vi "HFRR ADV v026 new software.vi"() -> ()   [LabVIEW 2025] (continued)
                n1899 = local read "string1"() -> (w2377:string)
              }
              frame True {
                n1900 = local read "String Indicator 4"() -> (w2378:string)
              }
            }
            n1901 = local read "string1 3"() -> (w2275:string)
            n1902 = String To Path(string=w2231) -> (path=w2362:path)
            n1903 = String To Path(string=w2275) -> (path=w2373:path)
            n1904 = local read "Numeric 12"() -> (w2359:i32)
            n1905 = local read "Numeric 8"() -> (w2361:i32)
            n1906 = local read "string1 2"() -> (w2276:string)
            n1907 = local read "string1 4"() -> (w2274:string)
            n1908 = Open/Create/Replace File "Open File"(file path (use dialog)=w2362) -> (refnum out=w2376:refnum<file>, error out=w2375:errorcluster)  [unwired: 5 in, 1 out]
            n1909 = Open/Create/Replace File "Open File"(file path (use dialog)=w2373) -> (refnum out=w2369:refnum<file>, error out=w2370:errorcluster)  [unwired: 5 in, 1 out]
            n1910 = for {
              N: w2361 -> [_]
              tunnel: w2376 -> [w2524]
              tunnel: w2375 -> [w2523]
              tunnel: [w2513] -> w2288 mode=indexing
              tunnel: [w2511] -> w2345 mode=indexing
              tunnel: [w2512] -> w2340 mode=indexing
              tunnel: w2357 -> [_]
              tunnel: [w2505] -> w2342 mode=indexing
              tunnel: [w2501] -> w2311 mode=indexing
              tunnel: [w2497] -> w2286 mode=indexing
              tunnel: [w2493] -> w2267 mode=indexing
              tunnel: [w2488] -> w2227 mode=indexing
              (unwired) TRUE ("line mode (F)")
              # "freq"
              # "Stroke"
              # "Time"
              # "CoF"
              # "Humidity"
              # "Temp"
              # "Air Temp"
              # "ECR"
              n1911 = Read from Text File "Read File"(file (use dialog)=w2524, error in=w2523) -> (text=w2489:string)  [unwired: 2 in, 3 out]
              n1912 = local write "String 6"(w2489) -> ()
              n1913 = String Subset(string=w2489, offset (0)=0, length (rest)=14 ("length (rest)")) -> (substring=w2517:string)
              n1914 = String Subset(string=w2489, offset (0)=35, length (rest)=9 ("length (rest)")) -> (substring=w2514:string)
              n1915 = String Subset(string=w2489, offset (0)=15, length (rest)=9 ("length (rest)")) -> (substring=w2520:string)
              n1916 = Fract/Exp String To Number(string=w2517) -> (number=w2513:dbl)  [unwired: 3 in, 1 out]
              n1917 = Fract/Exp String To Number(string=w2514) -> (number=w2512:dbl)  [unwired: 3 in, 1 out]
              n1918 = Fract/Exp String To Number(string=w2520) -> (number=w2511:dbl)  [unwired: 3 in, 1 out]
              n1919 = String Subset(string=w2489, offset (0)=85, length (rest)=9 ("length (rest)")) -> (substring=w2490:string)
              n1920 = String Subset(string=w2489, offset (0)=25, length (rest)=9 ("length (rest)")) -> (substring=w2496:string)
              n1921 = String Subset(string=w2489, offset (0)=55, length (rest)=9 ("length (rest)")) -> (substring=w2498:string)
              n1922 = String Subset(string=w2489, offset (0)=45, length (rest)=9 ("length (rest)")) -> (substring=w2504:string)
              n1923 = String Subset(string=w2489, offset (0)=65, length (rest)=9 ("length (rest)")) -> (substring=w2510:string)
              n1924 = Fract/Exp String To Number(string=w2496) -> (number=w2493:dbl)  [unwired: 3 in, 1 out]
              n1925 = Fract/Exp String To Number(string=w2490) -> (number=w2488:dbl)  [unwired: 3 in, 1 out]
              n1926 = Fract/Exp String To Number(string=w2498) -> (number=w2497:dbl)  [unwired: 3 in, 1 out]
              n1927 = Fract/Exp String To Number(string=w2504) -> (number=w2501:dbl)  [unwired: 3 in, 1 out]
              n1928 = Fract/Exp String To Number(string=w2510) -> (number=w2507:dbl)  [unwired: 3 in, 1 out]
              n1929 = Add(x=w2507, y=0.0) -> (x+y=w2505:dbl)
            }
            n1930 = for {
              N: w2359 -> [_]
              tunnel: w2370 -> [w2450]
              tunnel: w2369 -> [w2449]
              tunnel: [w2439] -> w2328 mode=indexing
              tunnel: [w2437] -> w2326 mode=indexing
              tunnel: [w2438] -> w2322 mode=indexing
              tunnel: w2357 -> [_]
              tunnel: [w2431] -> w2324 mode=indexing
              tunnel: [w2427] -> w2306 mode=indexing
              tunnel: [w2423] -> w2282 mode=indexing
              tunnel: [w2420] -> w2263 mode=indexing
              tunnel: [w2416] -> w2222 mode=indexing
              (unwired) 9 ("length (rest)")
              (unwired) 9 ("length (rest)")
              (unwired) TRUE ("line mode (F)")
              n1931 = Read from Text File "Read File"(file (use dialog)=w2449, error in=w2450) -> (text=w2417:string)  [unwired: 2 in, 3 out]
              n1932 = local write "String 8"(w2417) -> ()
              n1933 = String Subset(string=w2417, offset (0)=85) -> (substring=w2419:string)  [unwired: 1 in]
              n1934 = String Subset(string=w2417, offset (0)=35, length (rest)=9 ("length (rest)")) -> (substring=w2440:string)
              n1935 = String Subset(string=w2417, offset (0)=55, length (rest)=9 ("length (rest)")) -> (substring=w2425:string)
              n1936 = String Subset(string=w2417, offset (0)=25) -> (substring=w2421:string)  [unwired: 1 in]
              n1937 = String Subset(string=w2417, offset (0)=15, length (rest)=9 ("length (rest)")) -> (substring=w2446:string)
              n1938 = String Subset(string=w2417, offset (0)=0, length (rest)=14 ("length (rest)")) -> (substring=w2443:string)
              n1939 = String Subset(string=w2417, offset (0)=45, length (rest)=9 ("length (rest)")) -> (substring=w2430:string)
              n1940 = String Subset(string=w2417, offset (0)=65, length (rest)=9 ("length (rest)")) -> (substring=w2436:string)
              n1941 = Fract/Exp String To Number(string=w2419) -> (number=w2416:dbl)  [unwired: 3 in, 1 out]
              n1942 = Fract/Exp String To Number(string=w2440) -> (number=w2438:dbl)  [unwired: 3 in, 1 out]
              n1943 = Fract/Exp String To Number(string=w2425) -> (number=w2423:dbl)  [unwired: 3 in, 1 out]
              n1944 = Fract/Exp String To Number(string=w2421) -> (number=w2420:dbl)  [unwired: 3 in, 1 out]
              n1945 = Fract/Exp String To Number(string=w2446) -> (number=w2437:dbl)  [unwired: 3 in, 1 out]
              n1946 = Fract/Exp String To Number(string=w2443) -> (number=w2439:dbl)  [unwired: 3 in, 1 out]
              n1947 = Fract/Exp String To Number(string=w2430) -> (number=w2427:dbl)  [unwired: 3 in, 1 out]
              n1948 = Fract/Exp String To Number(string=w2436) -> (number=w2433:dbl)  [unwired: 3 in, 1 out]
              n1949 = Add(x=w2433, y=0.0) -> (x+y=w2431:dbl)
            }
            n1950 = String To Path(string=w2276) -> (path=w2374:path)
            n1951 = String To Path(string=w2274) -> (path=w2368:path)
            n1952 = local read "Numeric 11"() -> (w2358:i32)
            n1953 = local read "Numeric 13"() -> (w2360:i32)
            n1954 = Open/Create/Replace File "Open File"(file path (use dialog)=w2374) -> (refnum out=w2372:refnum<file>, error out=w2371:errorcluster)  [unwired: 5 in, 1 out]
            n1955 = Open/Create/Replace File "Open File"(file path (use dialog)=w2368) -> (refnum out=w2367:refnum<file>, error out=w2366:errorcluster)  [unwired: 5 in, 1 out]
            n1956 = for {
              N: w2358 -> [_]
              tunnel: w2372 -> [w2487]
              tunnel: w2371 -> [w2486]
              tunnel: [w2476] -> w2338 mode=indexing
              tunnel: [w2474] -> w2336 mode=indexing
              tunnel: [w2475] -> w2331 mode=indexing
              tunnel: w2357 -> [_]
              tunnel: [w2468] -> w2333 mode=indexing
              tunnel: [w2464] -> w2309 mode=indexing
              tunnel: [w2460] -> w2284 mode=indexing
              tunnel: [w2456] -> w2265 mode=indexing
              tunnel: [w2451] -> w2223 mode=indexing
              (unwired) TRUE ("line mode (F)")
              n1957 = Read from Text File "Read File"(file (use dialog)=w2487, error in=w2486) -> (text=w2452:string)  [unwired: 2 in, 3 out]
              n1958 = local write "String 7"(w2452) -> ()
              n1959 = String Subset(string=w2452, offset (0)=85, length (rest)=9 ("length (rest)")) -> (substring=w2455:string)
              n1960 = String Subset(string=w2452, offset (0)=35, length (rest)=9 ("length (rest)")) -> (substring=w2477:string)
              n1961 = String Subset(string=w2452, offset (0)=55, length (rest)=9 ("length (rest)")) -> (substring=w2463:string)
              n1962 = String Subset(string=w2452, offset (0)=25, length (rest)=9 ("length (rest)")) -> (substring=w2457:string)
              n1963 = String Subset(string=w2452, offset (0)=45, length (rest)=9 ("length (rest)")) -> (substring=w2465:string)
              n1964 = String Subset(string=w2452, offset (0)=0, length (rest)=14 ("length (rest)")) -> (substring=w2480:string)
              n1965 = String Subset(string=w2452, offset (0)=15, length (rest)=9 ("length (rest)")) -> (substring=w2483:string)
              n1966 = String Subset(string=w2452, offset (0)=65, length (rest)=9 ("length (rest)")) -> (substring=w2469:string)
              n1967 = Fract/Exp String To Number(string=w2455) -> (number=w2451:dbl)  [unwired: 3 in, 1 out]
              n1968 = Fract/Exp String To Number(string=w2477) -> (number=w2475:dbl)  [unwired: 3 in, 1 out]
              n1969 = Fract/Exp String To Number(string=w2463) -> (number=w2460:dbl)  [unwired: 3 in, 1 out]
              n1970 = Fract/Exp String To Number(string=w2457) -> (number=w2456:dbl)  [unwired: 3 in, 1 out]
              n1971 = Fract/Exp String To Number(string=w2465) -> (number=w2464:dbl)  [unwired: 3 in, 1 out]
              n1972 = Fract/Exp String To Number(string=w2480) -> (number=w2476:dbl)  [unwired: 3 in, 1 out]
              n1973 = Fract/Exp String To Number(string=w2483) -> (number=w2474:dbl)  [unwired: 3 in, 1 out]
              n1974 = Fract/Exp String To Number(string=w2469) -> (number=w2472:dbl)  [unwired: 3 in, 1 out]
              n1975 = Add(x=w2472, y=0.0) -> (x+y=w2468:dbl)
            }
            n1976 = for {
              N: w2360 -> [_]
              tunnel: w2367 -> [w2415]
              tunnel: w2366 -> [w2414]
              tunnel: [w2404] -> w2320 mode=indexing
              tunnel: [w2403] -> w2313 mode=indexing
              tunnel: w2357 -> [_]
              tunnel: [w2392] -> w2318 mode=indexing
              tunnel: [w2397] -> w2315 mode=indexing
              tunnel: [w2393] -> w2305 mode=indexing
              tunnel: [w2388] -> w2280 mode=indexing
              tunnel: [w2384] -> w2261 mode=indexing
              tunnel: [w2379] -> w2221 mode=indexing
              (unwired) 1.0 ("x")
              (unwired) TRUE ("line mode (F)")
              n1977 = Read from Text File "Read File"(file (use dialog)=w2415, error in=w2414) -> (text=w2380:string)  [unwired: 2 in, 3 out]
              n1978 = local write "String 12"(w2380) -> ()
              n1979 = String Subset(string=w2380, offset (0)=85, length (rest)=9 ("length (rest)")) -> (substring=w2382:string)
              n1980 = String Subset(string=w2380, offset (0)=35, length (rest)=9 ("length (rest)")) -> (substring=w2405:string)
              n1981 = String Subset(string=w2380, offset (0)=55, length (rest)=9 ("length (rest)")) -> (substring=w2390:string)
              n1982 = String Subset(string=w2380, offset (0)=25, length (rest)=9 ("length (rest)")) -> (substring=w2386:string)
              n1983 = String Subset(string=w2380, offset (0)=45, length (rest)=9 ("length (rest)")) -> (substring=w2395:string)
              n1984 = String Subset(string=w2380, offset (0)=15, length (rest)=9 ("length (rest)")) -> (substring=w2411:string)
              n1985 = String Subset(string=w2380, offset (0)=0, length (rest)=14 ("length (rest)")) -> (substring=w2408:string)
              n1986 = String Subset(string=w2380, offset (0)=65, length (rest)=9 ("length (rest)")) -> (substring=w2398:string)
              n1987 = Fract/Exp String To Number(string=w2382) -> (number=w2379:dbl)  [unwired: 3 in, 1 out]
              n1988 = Fract/Exp String To Number(string=w2405) -> (number=w2403:dbl)  [unwired: 3 in, 1 out]
              n1989 = Fract/Exp String To Number(string=w2390) -> (number=w2388:dbl)  [unwired: 3 in, 1 out]
              n1990 = Fract/Exp String To Number(string=w2386) -> (number=w2384:dbl)  [unwired: 3 in, 1 out]
              n1991 = Fract/Exp String To Number(string=w2395) -> (number=w2393:dbl)  [unwired: 3 in, 1 out]
              n1992 = Fract/Exp String To Number(string=w2411) -> (number=w2392:dbl)  [unwired: 3 in, 1 out]
              n1993 = Fract/Exp String To Number(string=w2408) -> (number=w2404:dbl)  [unwired: 3 in, 1 out]
              n1994 = Fract/Exp String To Number(string=w2398) -> (number=w2401:dbl)  [unwired: 3 in, 1 out]
              n1995 = Add(x=w2401, y=0.0) -> (x+y=w2397:dbl)
            }
            n1996 = Delete From Array(array=w2263, index=0) -> (array with subset deleted=w2236:dbl[])  [unwired: 1 in, 1 out]
            n1997 = Delete From Array(array=w2326, index=0) -> (array with subset deleted=w2299:dbl[])  [unwired: 1 in, 1 out]
            n1998 = Delete From Array(array=w2306, index=0) -> (array with subset deleted=w2294:dbl[])  [unwired: 1 in, 1 out]
            n1999 = Delete From Array(array=w2324, index=0) -> (array with subset deleted=w2325:dbl[])  [unwired: 1 in, 1 out]
            n2000 = call-poly <vilib>:"Mean.vi"("X"=w2236) -> ("mean"=→"КОФ2 4":dbl)  [unwired: 1 out]
            n2001 = call-poly <vilib>:"Mean.vi"("X"=w2299) -> ("mean"=→"КОФ3":dbl)  [unwired: 1 out]
            n2002 = call-poly <vilib>:"Mean.vi"("X"=w2294) -> ("mean"=→"CP3":dbl)  [unwired: 1 out]
            n2003 = Delete From Array(array=w2288, index=0) -> (array with subset deleted=w2215:dbl[])  [unwired: 1 in, 1 out]
            n2004 = Delete From Array(array=w2227, index=0) -> (array with subset deleted=w2214:dbl[])  [unwired: 1 in, 1 out]
            n2005 = Delete From Array(array=w2267, index=0) -> (array with subset deleted=w2238:dbl[])  [unwired: 1 in, 1 out]
            n2006 = Delete From Array(array=w2345, index=0) -> (array with subset deleted=w2300:dbl[])  [unwired: 1 in, 1 out]
            n2007 = Delete From Array(array=w2311, index=0) -> (array with subset deleted=w2296:dbl[])  [unwired: 1 in, 1 out]
            "array w/ subset deleted" <- w2296
            n2008 = Delete From Array(array=w2342, index=0) -> (array with subset deleted=w2343:dbl[])  [unwired: 1 in, 1 out]
            n2009 = call-poly <vilib>:"Mean.vi"("X"=w2238) -> ("mean"=→"КОФ2 2":dbl)  [unwired: 1 out]
            n2010 = call-poly <vilib>:"Mean.vi"("X"=w2300) -> ("mean"=→"КОФ1":dbl)  [unwired: 1 out]
            n2011 = Bundle "Bundle"(w2215, w2214) -> (w2220:cluster{dbl[], dbl[]})  [unwired: 1 in]
            n2012 = Bundle "Bundle"(w2215, w2343) -> (w2207:cluster{dbl[], dbl[]})  [unwired: 1 in]
            n2013 = Delete From Array(array=w2222, index=0) -> (array with subset deleted=w2210:dbl[])  [unwired: 1 in, 1 out]
            n2014 = Delete From Array(array=w2223, index=0) -> (array with subset deleted=w2212:dbl[])  [unwired: 1 in, 1 out]
            n2015 = Delete From Array(array=w2333, index=0) -> (array with subset deleted=w2334:dbl[])  [unwired: 1 in, 1 out]
            n2016 = Delete From Array(array=w2221, index=0) -> (array with subset deleted=w2208:dbl[])  [unwired: 1 in, 1 out]
            n2017 = Delete From Array(array=w2315, index=0) -> (array with subset deleted=w2316:dbl[])  [unwired: 1 in, 1 out]
            n2018 = Delete From Array(array=w2340, index=0) -> (array with subset deleted=w2246:dbl[])  [unwired: 1 in, 1 out]
            n2019 = Delete From Array(array=w2286, index=0) -> (array with subset deleted=w2242:dbl[])  [unwired: 1 in, 1 out]
            n2020 = Delete From Array(array=w2322, index=0) -> (array with subset deleted=w2244:dbl[])  [unwired: 1 in, 1 out]
            n2021 = Delete From Array(array=w2282, index=0) -> (array with subset deleted=w2240:dbl[])  [unwired: 1 in, 1 out]
            n2022 = Delete From Array(array=w2331, index=0) -> (array with subset deleted=w2245:dbl[])  [unwired: 1 in, 1 out]
            n2023 = Delete From Array(array=w2284, index=0) -> (array with subset deleted=w2241:dbl[])  [unwired: 1 in, 1 out]
            n2024 = Delete From Array(array=w2265, index=0) -> (array with subset deleted=w2237:dbl[])  [unwired: 1 in, 1 out]
            n2025 = Delete From Array(array=w2309, index=0) -> (array with subset deleted=w2295:dbl[])  [unwired: 1 in, 1 out]
            n2026 = Delete From Array(array=w2336, index=0) -> (array with subset deleted=w2297:dbl[])  [unwired: 1 in, 1 out]
            n2027 = Delete From Array(array=w2313, index=0) -> (array with subset deleted=w2243:dbl[])  [unwired: 1 in, 1 out]
            n2028 = Delete From Array(array=w2280, index=0) -> (array with subset deleted=w2239:dbl[])  [unwired: 1 in, 1 out]
            n2029 = Delete From Array(array=w2261, index=0) -> (array with subset deleted=w2235:dbl[])  [unwired: 1 in, 1 out]
            n2030 = Delete From Array(array=w2305, index=0) -> (array with subset deleted=w2293:dbl[])  [unwired: 1 in, 1 out]
            n2031 = Delete From Array(array=w2318, index=0) -> (array with subset deleted=w2298:dbl[])  [unwired: 1 in, 1 out]
            n2032 = Delete From Array(array=w2328, index=0) -> (array with subset deleted=w2211:dbl[])  [unwired: 1 in, 1 out]
            n2033 = Delete From Array(array=w2338, index=0) -> (array with subset deleted=w2213:dbl[])  [unwired: 1 in, 1 out]
            n2034 = Delete From Array(array=w2320, index=0) -> (array with subset deleted=w2209:dbl[])  [unwired: 1 in, 1 out]
            n2035 = Bundle "Bundle"(w2215, w2246) -> (w2233:cluster{dbl[], dbl[]})  [unwired: 1 in]
            n2036 = Bundle "Bundle"(w2215, w2300) -> (w2234:cluster{dbl[], dbl[]})  [unwired: 1 in]
            n2037 = Bundle "Bundle"(w2246, w2242) -> (w2248:cluster{dbl[], dbl[]})  [unwired: 1 in]
            n2038 = Bundle "Bundle"(w2211, w2210) -> (w2218:cluster{dbl[], dbl[]})  [unwired: 1 in]
            n2039 = Bundle "Bundle"(w2244, w2240) -> (w2250:cluster{dbl[], dbl[]})  [unwired: 1 in]
            n2040 = Bundle "Bundle"(w2211, w2244) -> (w2354:cluster{dbl[], dbl[]})  [unwired: 1 in]
            n2041 = Bundle "Bundle"(w2211, w2240) -> (w2278:cluster{dbl[], dbl[]})  [unwired: 1 in]
            n2042 = Bundle "Bundle"(w2211, w2299) -> (w2364:cluster{dbl[], dbl[]})  [unwired: 1 in]
            n2043 = Bundle "Bundle"(w2211, w2294) -> (w2302:cluster{dbl[], dbl[]})  [unwired: 1 in]
            n2044 = Bundle "Bundle"(w2211, w2325) -> (w2349:cluster{dbl[], dbl[]})  [unwired: 1 in]
            n2045 = Bundle "Bundle"(w2245, w2241) -> (w2249:cluster{dbl[], dbl[]})  [unwired: 1 in]
            n2046 = Bundle "Bundle"(w2213, w2212) -> (w2219:cluster{dbl[], dbl[]})  [unwired: 1 in]
            n2047 = Bundle "Bundle"(w2213, w2245) -> (w2356:cluster{dbl[], dbl[]})  [unwired: 1 in]
            n2048 = Bundle "Bundle"(w2213, w2241) -> (w2279:cluster{dbl[], dbl[]})  [unwired: 1 in]
            n2049 = Bundle "Bundle"(w2213, w2295) -> (w2303:cluster{dbl[], dbl[]})  [unwired: 1 in]
            n2050 = Bundle "Bundle"(w2213, w2297) -> (w2365:cluster{dbl[], dbl[]})  [unwired: 1 in]
            n2051 = Bundle "Bundle"(w2213, w2334) -> (w2347:cluster{dbl[], dbl[]})  [unwired: 1 in]
            n2052 = Bundle "Bundle"(w2243, w2239) -> (w2251:cluster{dbl[], dbl[]})  [unwired: 1 in]
            n2053 = Bundle "Bundle"(w2209, w2208) -> (w2217:cluster{dbl[], dbl[]})  [unwired: 1 in]
            n2054 = Bundle "Bundle"(w2209, w2243) -> (w2355:cluster{dbl[], dbl[]})  [unwired: 1 in]
            n2055 = Bundle "Bundle"(w2209, w2239) -> (w2277:cluster{dbl[], dbl[]})  [unwired: 1 in]
            n2056 = Bundle "Bundle"(w2209, w2293) -> (w2301:cluster{dbl[], dbl[]})  [unwired: 1 in]
            n2057 = Bundle "Bundle"(w2209, w2298) -> (w2363:cluster{dbl[], dbl[]})  [unwired: 1 in]
            n2058 = Bundle "Bundle"(w2209, w2316) -> (w2348:cluster{dbl[], dbl[]})  [unwired: 1 in]
            n2059 = call-poly <vilib>:"Mean.vi"("X"=w2296) -> ("mean"=→"CP1":dbl)  [unwired: 1 out]
            n2060 = call-poly <vilib>:"Mean.vi"("X"=w2237) -> ("mean"=→"КОФ2 3":dbl)  [unwired: 1 out]
            n2061 = call-poly <vilib>:"Mean.vi"("X"=w2295) -> ("mean"=→"CP2":dbl)  [unwired: 1 out]
            n2062 = call-poly <vilib>:"Mean.vi"("X"=w2297) -> ("mean"=→"КОФ2":dbl)  [unwired: 1 out]
            n2063 = call-poly <vilib>:"Mean.vi"("X"=w2235) -> ("mean"=→"КОФ2 5":dbl)  [unwired: 1 out]
            n2064 = call-poly <vilib>:"Mean.vi"("X"=w2293) -> ("mean"=→"CP4":dbl)  [unwired: 1 out]
            n2065 = call-poly <vilib>:"Mean.vi"("X"=w2298) -> ("mean"=→"КОФ4":dbl)  [unwired: 1 out]
            n2066 = Bundle "Bundle"(w2215, w2242) -> (w2206:cluster{dbl[], dbl[]})  [unwired: 1 in]
            n2067 = Bundle "Bundle"(w2215, w2296) -> (w2229:cluster{dbl[], dbl[]})  [unwired: 1 in]
            n2068 = Build Array "Build Array"(w2206, w2229) -> (w2232:cluster{dbl[], dbl[]}[])
            "XY Graph 17" <- w2232
            n2069 = Build Array "Build Array"(w2220, w2219, w2218, w2217) -> (→"Frequency ( Hz )":cluster{dbl[], dbl[]}[])
            n2070 = Build Array "Build Array"(w2248, w2249, w2250, w2251) -> (→"Air Temp ( °C ) vs Humidity ( % RH )":cluster{dbl[], dbl[]}[])
            n2071 = Build Array "Build Array"(w2233, w2356, w2354, w2355) -> (→"Air Temperature  ( °C )":cluster{dbl[], dbl[]}[])
            n2072 = Build Array "Build Array"(w2206, w2279, w2278, w2277) -> (→"Humidity ( %RH )":cluster{dbl[], dbl[]}[])
            n2073 = Build Array "Build Array"(w2234, w2365, w2364, w2363) -> (→"Coefficient Of Friction":cluster{dbl[], dbl[]}[])
            n2074 = Build Array "Build Array"(w2229, w2303, w2302, w2301) -> (→"Sample Temperature ( °C )":cluster{dbl[], dbl[]}[])
            n2075 = Build Array "Build Array"(w2207, w2347, w2349, w2348) -> (→"XY Graph 13":cluster{dbl[], dbl[]}[])
            n2076 = Bundle "Bundle"(w2215, w2238) -> (w2260:cluster{dbl[], dbl[]})  [unwired: 1 in]
            n2077 = Bundle "Bundle"(w2211, w2236) -> (w2258:cluster{dbl[], dbl[]})  [unwired: 1 in]
            n2078 = Bundle "Bundle"(w2213, w2237) -> (w2259:cluster{dbl[], dbl[]})  [unwired: 1 in]
            n2079 = Bundle "Bundle"(w2209, w2235) -> (w2257:cluster{dbl[], dbl[]})  [unwired: 1 in]
            n2080 = Build Array "Build Array"(w2260, w2259, w2258, w2257) -> (→"Stroke ( mm )":cluster{dbl[], dbl[]}[])
            n2081 = local write "XY Graph 16"(w2232) -> ()
          }
          frame #2 {
          }
          frame #3 {
            n2082 = local write "Numeric 8"(0 ("Numeric 8")) -> ()
            n2083 = local write "Numeric 11"(0 ("Numeric 11")) -> ()
            n2084 = local write "Numeric 12"(0 ("Numeric 12")) -> ()
            n2085 = local write "Numeric 13"(0 ("Numeric 13")) -> ()
            n2086 = property on="OPEN" class="Bool (strict)"("Visible"=TRUE) -> ()  [unwired: 2 in, 2 out]
            n2087 = local read "String Control 2"() -> (w2532:string)
            n2088 = local read "String Control 4"() -> (w2531:string)
            n2089 = local read "String Control 6"() -> (w2530:string)
            n2090 = local read "String Control 8"() -> (w2529:string)
            n2091 = Match Pattern(string=w2532, regular expression="Samples / cycle :- ") -> (after substring=w2546:string)  [unwired: 1 in, 3 out]
            n2092 = Match Pattern(string=w2532, regular expression="Frequency :- ") -> (after substring=w2565:string)  [unwired: 1 in, 3 out]
            n2093 = Match Pattern(string=w2531, regular expression="Samples / cycle :- ") -> (after substring=w2542:string)  [unwired: 1 in, 3 out]
            n2094 = Match Pattern(string=w2531, regular expression="Frequency :- ") -> (after substring=w2560:string)  [unwired: 1 in, 3 out]
            n2095 = Match Pattern(string=w2530, regular expression="Samples / cycle :- ") -> (after substring=w2538:string)  [unwired: 1 in, 3 out]
            n2096 = Match Pattern(string=w2530, regular expression="Frequency :- ") -> (after substring=w2555:string)  [unwired: 1 in, 3 out]
            n2097 = Match Pattern(string=w2529, regular expression="Samples / cycle :- ") -> (after substring=w2534:string)  [unwired: 1 in, 3 out]
            n2098 = Match Pattern(string=w2529, regular expression="Frequency :- ") -> (after substring=w2550:string)  [unwired: 1 in, 3 out]
            n2099 = String Subset(string=w2546, length (rest)=6 ("length (rest)")) -> (substring=w2548:string)  [unwired: 1 in]
            n2100 = String Subset(string=w2565, length (rest)=9 ("length (rest)")) -> (substring=w2567:string)  [unwired: 1 in]
            n2101 = String Subset(string=w2542, length (rest)=6 ("length (rest)")) -> (substring=w2544:string)  [unwired: 1 in]
            n2102 = String Subset(string=w2560, length (rest)=9 ("length (rest)")) -> (substring=w2562:string)  [unwired: 1 in]
            n2103 = String Subset(string=w2538, length (rest)=6 ("length (rest)")) -> (substring=w2540:string)  [unwired: 1 in]
            n2104 = String Subset(string=w2555, length (rest)=9 ("length (rest)")) -> (substring=w2557:string)  [unwired: 1 in]
            n2105 = String Subset(string=w2534, length (rest)=6 ("length (rest)")) -> (substring=w2536:string)  [unwired: 1 in]
            n2106 = String Subset(string=w2550, length (rest)=9 ("length (rest)")) -> (substring=w2552:string)  [unwired: 1 in]
            n2107 = Fract/Exp String To Number(string=w2548) -> (number=w2528:dbl)  [unwired: 3 in, 1 out]
            n2108 = Fract/Exp String To Number(string=w2567) -> (number=w2568:dbl)  [unwired: 3 in, 1 out]
            n2109 = Fract/Exp String To Number(string=w2544) -> (number=w2527:dbl)  [unwired: 3 in, 1 out]
            n2110 = Fract/Exp String To Number(string=w2562) -> (number=w2563:dbl)  [unwired: 3 in, 1 out]
            n2111 = Fract/Exp String To Number(string=w2540) -> (number=w2526:dbl)  [unwired: 3 in, 1 out]
            n2112 = Fract/Exp String To Number(string=w2557) -> (number=w2558:dbl)  [unwired: 3 in, 1 out]
            n2113 = Fract/Exp String To Number(string=w2536) -> (number=w2525:dbl)  [unwired: 3 in, 1 out]
            n2114 = Fract/Exp String To Number(string=w2552) -> (number=w2553:dbl)  [unwired: 3 in, 1 out]
            n2115 = local write "sample1"(w2528) -> ()
            n2116 = local write "freq1"(w2568) -> ()
            n2117 = local write "sample2"(w2527) -> ()
            n2118 = local write "freq2"(w2563) -> ()
            n2119 = local write "sample3"(w2526) -> ()
            n2120 = local write "freq3"(w2558) -> ()
            n2121 = local write "sample4"(w2525) -> ()
            n2122 = local write "freq 4"(w2553) -> ()
          }
        }
      }
    }
    n2123 = case shown="True" w2126 {
      selector: w2126 -> [_ w2145]
      frame False {
      }
      frame True {
        n2124 = Not(x=w2145) -> (.not. x?=w2141:bool)
        n2125 = local write "service 3"(w2141) -> ()
        n2126 = local write "OPEN 6"(w2141) -> ()
        n2127 = call <vilib>:"System Exec.vi"("wait until completion? (T)"=TRUE, "command line"="C:\\LAB-IQ\\Scar View.exe") -> ("error out"=→"error out 5":errorcluster)  [unwired: 6 in, 3 out]
      }
    }
    n2128 = case shown="\"Acquire\", Default" w2135 {
      frame "Acquire", Default {
        # "Elapsed time\ncof\nstroke\nAir temp\nTemp\nHumidity"
        n2129 = disable-structure shown="Disabled" {
          frame Disabled {
            n2130 = local read "Flag"() -> (w2844:dbl)
            n2131 = local read "RUN"() -> (w2841:bool)
            n2132 = Not(x=w2841) -> (.not. x?=w2840:bool)
            n2133 = Equal?(x=w2844, y=10.0) -> (x = y?=w2842:bool)
            n2134 = And(x=w2842, y=w2840) -> (x .and. y?=w2839:bool)
            n2135 = case shown="True" w2839 {
              frame False {
              }
              frame True {
                w2845 = FALSE ("Heater Button")
                n2136 = local write "Humidity"(w2845) -> ()
                n2137 = local write "Heater Button"(w2845) -> ()
              }
            }
          }
          frame Enabled {
          }
        }
        n2138 = disable-structure shown="Disabled" {
          frame Disabled {
            n2139 = case shown="True" {
              selector: _ -> [_ _]
              frame False {
              }
              frame True {
                w2898 = TRUE ("Heater")
                n2140 = local write "Humidity"(w2898) -> ()
                n2141 = local write "Heater Button"(w2898) -> ()
                n2142 = local read "TEST STANDARD"() -> (w2901:T3)
                n2143 = local read "TEST STANDARD"() -> (w2896:T3)
                n2144 = Equal?(x=w2901, y=enum16{"ASTM D6079", "ISO 12156", "Custom"}."ISO 12156" ("Test Standard")) -> (x = y?=w2899:bool)
                n2145 = Equal?(x=w2896, y=enum16{"ASTM D6079", "ISO 12156", "Custom"}."ASTM D6079" ("Test Standard")) -> (x = y?=w2895:bool)
                n2146 = case shown="True" w2899 {
                  frame False {
                  }
                  frame True {
                    n2147 = local write "airtempflg"(FALSE ("airtempflg")) -> ()
                    n2148 = local write item#-1(TRUE ("Heater")) -> ()
                  }
                }
                n2149 = case shown="True" w2895 {
                  frame False {
                  }
                  frame True {
                    n2150 = local write "airtempflg"(TRUE ("airtempflg")) -> ()
                    n2151 = local write item#-1(FALSE ("Heater")) -> ()
                  }
                }
              }
            }
          }
          frame Enabled {
          }
        }
        n2152 = stacked-sequence {
          frame #0 {
            n2153 = case shown="True" "RST FF" {
              frame False {
              }
              frame True {
                w2915 = 0.0 ("X Scale.Range:Maximum")
                n2154 = property on="Frictional Force ( N )" class="WFChart (strict)"("XScale.Maximum"=600.0 ("X Scale.Range:Maximum"), "XScale.Minimum"=w2915, "YScale.Maximum"=10.0 ("Y Scale.Range:Maximum"), "YScale.Minimum"=w2915) -> ()  [unwired: 2 in, 2 out]
              }
            }
          }
          frame #1 {
            n2155 = case shown="True" "RST TEMP" {
              frame False {
              }
              frame True {
                n2156 = property on="Temperature ( Deg C )" class="WFChart (strict)"("XScale.Minimum"=0.0 ("X Scale.Range:Minimum"), "XScale.Maximum"=600.0 ("X Scale.Range:Maximum"), "YScale.Minimum"=0.0 ("Y Scale.Range:Minimum"), "YScale.Maximum"=100.0 ("Y Scale.Range:Maximum")) -> ()  [unwired: 2 in, 2 out]
              }
            }
          }
          frame #2 {
            n2157 = case shown="True" "RSTCOF" {
              frame False {
              }
              frame True {
                n2158 = property on="Coefficient of Friction" class="WFChart (strict)"("XScale.Minimum"=0.0 ("X Scale.Range:Minimum"), "XScale.Maximum"=600.0 ("X Scale.Range:Maximum"), "YScale.Maximum"=1.0 ("X Scale.Range:Minimum"), "YScale.Minimum"=0.0 ("X Scale.Range:Minimum")) -> ()  [unwired: 2 in, 2 out]
              }
            }
          }
          frame #3 {
            n2159 = case shown="True" "RSTCOF 2" {
              frame False {
              }
              frame True {
                (unwired) 100.0 ("Y Scale.Range:Maximum")
                (unwired) 0.0 ("Y Scale.Range:Minimum")
                (unwired) 600.0 ("X Scale.Range:Maximum")
                (unwired) 0.0 ("X Scale.Range:Minimum")
              }
            }
          }
          frame #4 {
            n2160 = case shown="True" "RSTCOF 3" {
              frame False {
              }
              frame True {
                n2161 = property on="Electrical Contact Resistance ( % )" class="WFChart (strict)"("XScale.Minimum"=0.0 ("X Scale.Range:Minimum"), "XScale.Maximum"=600.0 ("X Scale.Range:Maximum"), "YScale.Minimum"=0.0 ("Y Scale.Range:Minimum"), "YScale.Maximum"=100.0 ("Y Scale.Range:Maximum")) -> ()  [unwired: 2 in, 2 out]
              }
            }
          }
        }
        n2162 = local read "RUN"() -> (w2834:bool)
        n2163 = case shown="False" w2834 {
          frame False {
          }
          frame True {
          }
        }
        n2164 = local read "RUN"() -> (w2838:bool)
        n2165 = case shown="False" w2838 {
          tunnel: [FALSE ("TEST RUNNING") TRUE ("TEST RUNNING")] -> w2837
          frame False {
            w2934 = 0.0 ("Flag")
            n2166 = local write "Elapsed time"(0.0 ("elapsedtime")) -> ()
            n2167 = local write "Time Remaining"(w2934) -> ()
            n2168 = local write "Flag"(w2934) -> ()
            n2169 = local write "Remaining Time"(w2934) -> ()
          }
          frame True {
            n2170 = local write "Flag"(10.0 ("Flag")) -> ()
          }
        }
        n2171 = local read "AIR TEMP"() -> (w2832:dbl)
        n2172 = Greater Or Equal?(x=w2832, y=15.0) -> (x >= y?=w2833:bool)
        "powstat" <- w2833
        n2173 = case shown="True" "Save & Continue" {
          frame False {
          }
          frame True {
            n2174 = local read "USER ID"() -> (w3227:string)
            n2175 = local read "FILE"() -> (w3235:string)
            n2176 = String Length(string=w3235) -> (length=w3233:i32)
            n2177 = String Length(string=w3227) -> (length=w3230:i32)
            n2178 = Greater?(x=w3233, y=0) -> (0:w3232:bool)
            n2179 = Greater?(x=w3230, y=0) -> (0:w3229:bool)
            n2180 = And(x=w3232, y=w3229) -> (x .and. y?=w3228:bool)
            n2181 = case shown="True" w3228 {
              frame False {
                n2182 = stacked-sequence {
                  frame #0 {
                    n2183 = One Button Dialog(message="Please Enter a File Name and Operator ID to save data !", button name ("OK")="Ok") -> ()  [unwired: 1 out]
                  }
                  frame #1 {
                    n2184 = local write "Save & Continue"(FALSE ("OK Button")) -> ()
                  }
                }
                n2185 = local write "Save & Continue"(FALSE ("OK Button")) -> ()
              }
              frame True {
                n2186 = stacked-sequence {
                  frame #0 {
                    n2187 = local read "FILE"() -> (w3241:string)
                    n2188 = call "file check.vi"("file name in"=w3241) -> ("file name out"=w3240:string)  [unwired: 9 in, 1 out]
                    n2189 = call <vilib>:"Application Directory.vi"() -> ("Application Directory"=w3251:path)
                    n2190 = Build Path(base path=w3251, name or relative path="data") -> (appended path=w3250:path)
                    n2191 = call <vilib>:"Trim Whitespace.vi"("string"=w3240) -> ("trimmed string"=w3248:string)  [unwired: 1 in]
                    n2192 = call <vilib>:"Trim Whitespace.vi"("string"=w3240) -> ("trimmed string"=w3249:string)  [unwired: 1 in]
                    n2193 = List Folder(path=w3250) -> (folder names=w3246:string[])  [unwired: 3 in, 3 out]
                    n2194 = Match Pattern(string=w3248, regular expression="_(") -> (before substring=w3245:string)  [unwired: 1 in, 3 out]
                    n2195 = for {
                      tunnel: w3246 -> [w3260] mode=indexing
                      tunnel: w3245 -> [w3258]
                      shift-right: [w3256] -> w3243
                      shift-left: bool[] [] -> [w3257]
                      n2196 = Match Pattern(string=w3260, regular expression="_(") -> (before substring=w3259:string)  [unwired: 1 in, 3 out]
                      n2197 = Equal?(x=w3259, y=w3258) -> (x = y?=w3255:bool)
                      n2198 = case shown="True" w3255 {
                        tunnel: w3255 -> [_ w3263]
                        tunnel: w3257 -> [w3262 w3265]
                        tunnel: [w3262 w3264] -> w3256
                        frame False {
                        }
                        frame True {
                          n2199 = Insert Into Array(array=w3265, new element=w3263) -> (w3264:bool[])  [unwired: 1 in]
                        }
                      }
                    }
                    n2200 = Equal?(x=w3246, y=w3245) -> (x = y?=w3254:bool[])
                    n2201 = Or Array Elements(Boolean array=w3254) -> (logical OR=w3253:bool)
                    n2202 = Array Size(array=w3243) -> (size(s)=w3242:i32)
                    n2203 = case shown="True" w3253 {
                      tunnel: w3249 -> [_ w3273]
                      tunnel: w3242 -> [_ w3266]
                      frame False {
                      }
                      frame True {
                        n2204 = Number To Decimal String(number=w3266) -> (decimal integer string=w3269:string)  [unwired: 1 in]
                        n2205 = Search/Split String(string=w3273, search string/char (-)="_(" ("regular expression")) -> (substring before match=w3271:string)  [unwired: 1 in, 2 out]
                        n2206 = Concatenate Strings(w3271, "_(" ("regular expression"), w3269, ")" ("regular expression")) -> (w3267:string)
                        n2207 = local write "FILE"(w3267) -> ()
                      }
                    }
                  }
                  frame #1 {
                    w3276 = 0.0
                    w3289 = cluster{"y":dbl, dbl, "y":dbl}[] [] ("History Data")
                    w3290 = FALSE ("Heater Button")
                    (unwired) ")!" ("string")
                    (unwired) ")" ("string")
                    w3288 = dbl[] [] ("History Data")
                    w3294 = "\r"
                    # "C:\\WinDucom\\Data\\"
                    # "C:\\LAB-IQ-NXT\\data"
                    n2208 = local write "Humidity ( %RH )"(w3276) -> ()
                    n2209 = local write "Frequency ( Hz )"(w3276) -> ()
                    n2210 = local write "Stroke 3"(w3276) -> ()
                    n2211 = local write "speedop"(0.0 ("PIDclk 2")) -> ()
                    n2212 = local write "Set Temp 2"(65.0 ("Set Temp 2")) -> ()
                    n2213 = local write "AIR TEMP"(w3276) -> ()
                    n2214 = local write "clk"(0.0 ("clk")) -> ()
                    n2215 = local write "Stroke 4"(w3276) -> ()
                    n2216 = local write "COF 2"(w3276) -> ()
                    n2217 = local write "TEMP"(w3276) -> ()
                    n2218 = local write "ecr 3"(w3276) -> ()
                    n2219 = local write "FF 3"(w3276) -> ()
                    n2220 = local write "FF 2"(w3276) -> ()
                    n2221 = property on="Humidity ( %RH )" class="WFChart (strict)"("History Data"=w3288) -> ()  [unwired: 2 in, 2 out]
                    n2222 = property on="Coefficient of Friction" class="WFChart (strict)"("History Data"=w3288) -> ()  [unwired: 2 in, 2 out]
                    n2223 = property on="Coefficient of Friction" class="WFChart (strict)"("History Data"=w3288) -> ()  [unwired: 2 in, 2 out]
                    n2224 = property on="Frictional Force ( N )" class="WFChart (strict)"("History Data"=w3288) -> ()  [unwired: 2 in, 2 out]
                    n2225 = property on="Electrical Contact Resistance ( % )" class="WFChart (strict)"("History Data"=w3288) -> ()  [unwired: 2 in, 2 out]
                    n2226 = property on="Electrical Contact Resistance ( % )" class="WFChart (strict)"("History Data"=w3288) -> ()  [unwired: 2 in, 2 out]
                    n2227 = property on="Temperature ( Deg C )" class="WFChart (strict)"("History Data"=w3288) -> ()  [unwired: 2 in, 2 out]
                    n2228 = property on="Frictional Force ( N )" class="WFChart (strict)"("History Data"=w3288) -> ()  [unwired: 2 in, 2 out]
                    n2229 = property on="Coefficient of Friction" class="WFChart (strict)"("History Data"=w3288) -> ()  [unwired: 2 in, 2 out]
                    n2230 = property on="Frictional Force ( N )" class="WFChart (strict)"("History Data"=w3288) -> ()  [unwired: 2 in, 2 out]
                    n2231 = property on="Electrical Contact Resistance ( % )" class="WFChart (strict)"("History Data"=w3288) -> ()  [unwired: 2 in, 2 out]
                    n2232 = property on="Temperature ( Deg C )" class="WFChart (strict)"("History Data"=w3288) -> ()  [unwired: 2 in, 2 out]
                    n2233 = property on="Humidity ( %RH )" class="WFChart (strict)"("History Data"=w3288) -> ()  [unwired: 2 in, 2 out]
                    n2234 = property on="Stroke ( mm )" class="WFChart (strict)"("History Data"=w3289) -> ()  [unwired: 2 in, 2 out]
                    n2235 = property on="Stroke ( mm )" class="WFChart (strict)"("History Data"=w3289) -> ()  [unwired: 2 in, 2 out]
                    n2236 = local write "Humidity"(w3290) -> ()
                    n2237 = local write "Heater Button"(w3290) -> ()
                    n2238 = local read "FILE"() -> (w3284:string)
                    n2239 = disable-structure shown="Enabled" {
                      disable-tunnel: [w3328 _] -> w3275
                      frame Enabled {
                        n2240 = local read "NORMAL LOAD"() -> (w3328:dbl)
                      }
                      frame Disabled {
                      }
                    }
                    n2241 = call "file check.vi"("file name in"=w3284) -> ("error out"=w3287:errorcluster, "file name out"=w3281:string)  [unwired: 9 in]
                    n2242 = call "FILE PATH CREATION.vi"("error in"=w3287, "FILE NAME :"=w3281) -> ("FILE OUT"=w3280:path)  [unwired: 8 in, 1 out]
                    n2243 = Concatenate Strings(w3281, ".dgf" ("Substring")) -> (w3286:string)
                    n2244 = Concatenate Strings(w3281, ".duf" ("Substring")) -> (w3282:string)
                    n2245 = Multiply(x=w3275, y=1.0) -> (x*y=w3307:dbl)
                    n2246 = Build Path(base path=w3280, name or relative path=w3286) -> (appended path=w3279:path)
                    n2247 = Build Path(base path=w3280, name or relative path=w3282) -> (appended path=w3278:path)
                    n2248 = Number To Fractional String(number=w3307, width (-)=i16 5, precision (6)=i16 2) -> (F-format string=w3315:string)  [unwired: 1 in]
                    n2249 = local read "tested by"() -> (w3274:string)
                    n2250 = local read "Fuel Discription :"() -> (w3303:string)
                    n2251 = local read "Batch Ref Num :"() -> (w3292:string)
                    n2252 = Get Date/Time String(date format (0)=enum16{"short", "long", "abbreviated"}."short") -> (date string=w3326:string, time string=w3323:string)  [unwired: 2 in]
                    n2253 = local read "Remarks :"() -> (w3302:string)
                    n2254 = Concatenate Strings("Load :- " ("Substring"), w3315, " grams ," ("Substring")) -> (w3314:string)
                    n2255 = local read "String 41"() -> (w3295:string)
                    n2256 = Concatenate Strings(w3303) -> (w3304:string)
                    n2257 = Concatenate Strings(w3292) -> (w3291:string)
                    n2258 = Concatenate Strings(w3274) -> (w3298:string)
                    n2259 = Concatenate Strings("(" ("Substring"), w3326, ")" ("Substring"), w3323) -> (w3297:string)
                    "concatenated string" <- w3297
                    n2260 = Concatenate Strings(w3302, "," ("string")) -> (w3301:string)
                    n2261 = Concatenate Strings("  TIME;      COF;       STROKE;     AIR TEMP;  TEMP;  HUMIDITY;  ECR; PID-OUT; FREQUENCY" ("Substring"), "\r") -> (w3310:string)
                    n2262 = Concatenate Strings(w3295, w3294, "Fuel Discription :-" ("Substring"), w3304, w3294, w3314, w3294, "Batch Ref Num :-" ("Substring"), w3291, w3294, " Remarks :- " ("Substring"), w3301, w3294, " Date :- " ("Substring"), w3297, w3294, "Tested By :-" ("Substring"), w3298) -> (w3308:string)
                    "REMARKS" <- w3308
                    n2263 = call <vilib>:"Write Characters To File.vi"("append to file? (new file:F)"=FALSE, "character string"=w3310, "file path (dialog if empty)"=w3279) -> ()  [unwired: 2 in, 1 out]
                    n2264 = call <vilib>:"Write Characters To File.vi"("append to file? (new file:F)"=FALSE, "character string"=w3308, "file path (dialog if empty)"=w3278) -> ()  [unwired: 2 in, 1 out]
                  }
                  frame #2 {
                    n2265 = local write "Cycles elapsed"(0 ("Cycles elapsed")) -> ()
                    n2266 = local write "cyclecount"(0 ("cyclecount")) -> ()
                    n2267 = local write "Save & Continue"(FALSE ("OK")) -> ()
                    n2268 = local write "autostrtflg"(TRUE ("autostrtflg")) -> ()
                    n2269 = local write "Save"(FALSE ("Save")) -> ()
                    n2270 = Get Date/Time In Seconds() -> (seconds since 1Jan1904=w3333:timestamp)
                    n2271 = To Double Precision Float(number=w3333) -> (double precision float=w3332:dbl)
                    n2272 = local write "acq timer"(w3332) -> ()
                    n2273 = One Button Dialog(message="Please ensure sample is mounted properly and machine is ready in all aspects for testing !", button name ("OK")="Ok") -> ()  [unwired: 1 out]
                  }
                  frame #3 {
                    n2274 = stacked-sequence {
                      frame #0 {
                        n2275 = local write "Main Dashboard Buttons"(T1."Dashboard" ("Main Dashboard Buttons")) -> ()
                        n2276 = local write "Main Tab"(T2."Acquire" ("Main Tab")) -> ()
                      }
                      frame #1 {
                        n2277 = local write "EVENT LOG"("" ("EVENT LOG")) -> ()
                      }
                      frame #2 {
                        n2278 = Wait (ms)(milliseconds to wait=u32 50) -> ()  [unwired: 1 out]
                      }
                      frame #3 {
                        n2279 = disable-structure shown="Disabled" {
                          frame Disabled {
                            n2280 = local read "EVENT LOG"() -> (w3345:string)
                            n2281 = call "Event Log.vi"("Content"="Test Details", "EVENT LOG"=w3345) -> ("EVENT LOG"=w3344:string)  [unwired: 8 in, 1 out]
                            n2282 = local write "EVENT LOG"(w3344) -> ()
                          }
                          frame Enabled {
                          }
                        }
                      }
                      frame #4 {
                        n2283 = Wait (ms)(milliseconds to wait=u32 50) -> ()  [unwired: 1 out]
                      }
                      frame #5 {
                        n2284 = local read "FILE"() -> (w3347:string)
                        n2285 = Concatenate Strings("File Name :" ("Content"), w3347) -> (w3348:string)
                        n2286 = local read "EVENT LOG"() -> (w3351:string)
                        n2287 = call "Event Log.vi"("Content"=w3348, "EVENT LOG"=w3351) -> ("EVENT LOG"=w3350:string)  [unwired: 8 in, 1 out]
                        n2288 = local write "EVENT LOG"(w3350) -> ()
                      }
                      frame #6 {
                        n2289 = Wait (ms)(milliseconds to wait=u32 50) -> ()  [unwired: 1 out]
                      }
                      frame #7 {
                        n2290 = local read "Batch Ref Num :"() -> (w3353:string)
                        n2291 = Concatenate Strings("Batch Ref No :" ("Content"), w3353) -> (w3354:string)
                        n2292 = local read "EVENT LOG"() -> (w3357:string)
                        n2293 = call "Event Log.vi"("Content"=w3354, "EVENT LOG"=w3357) -> ("EVENT LOG"=w3356:string)  [unwired: 8 in, 1 out]
                        n2294 = local write "EVENT LOG"(w3356) -> ()
                      }
                      frame #8 {
                        n2295 = Wait (ms)(milliseconds to wait=u32 50) -> ()  [unwired: 1 out]
                      }
                      frame #9 {
                        n2296 = local read "tested by"() -> (w3359:string)
                        n2297 = Concatenate Strings("Tested By :" ("Content"), w3359) -> (w3360:string)
                        n2298 = local read "EVENT LOG"() -> (w3363:string)
                        n2299 = call "Event Log.vi"("Content"=w3360, "EVENT LOG"=w3363) -> ("EVENT LOG"=w3362:string)  [unwired: 8 in, 1 out]
                        n2300 = local write "EVENT LOG"(w3362) -> ()
                      }
                      frame #10 {
                        n2301 = Wait (ms)(milliseconds to wait=u32 50) -> ()  [unwired: 1 out]
                      }
                      frame #11 {
                        n2302 = local read "TEST STANDARD"() -> (w3366:T3)
                        n2303 = case shown="\"ASTM D6079\", Default" w3366 {
                          tunnel: ["ASTM D6079" "ISO 12156" "CEC F-096-A-06" "Custom"] -> w3365
                          frame "ASTM D6079", Default {
                          }
                          frame "ISO 12156" {
                          }
                          frame "CEC F-096-A-06" {
                          }
                          frame "Custom" {
                          }
                        }
                        n2304 = Concatenate Strings("Test Standard :" ("Content"), w3365) -> (w3367:string)
                        n2305 = local read "EVENT LOG"() -> (w3370:string)
                        n2306 = call "Event Log.vi"("Content"=w3367, "EVENT LOG"=w3370) -> ("EVENT LOG"=w3369:string)  [unwired: 8 in, 1 out]
                        n2307 = local write "EVENT LOG"(w3369) -> ()
                      }
                      frame #12 {
                        n2308 = Wait (ms)(milliseconds to wait=u32 50) -> ()  [unwired: 1 out]
                      }
                      frame #13 {
                        n2309 = local read "Fuel Discription :"() -> (w3376:string)
                        n2310 = Concatenate Strings("Fuel Description :" ("Content"), w3376) -> (w3377:string)
                        n2311 = local read "EVENT LOG"() -> (w3380:string)
                        n2312 = call "Event Log.vi"("Content"=w3377, "EVENT LOG"=w3380) -> ("EVENT LOG"=w3379:string)  [unwired: 8 in, 1 out]
                        n2313 = local write "EVENT LOG"(w3379) -> ()
                      }
                      frame #14 {
                        n2314 = Wait (ms)(milliseconds to wait=u32 50) -> ()  [unwired: 1 out]
                      }
                      frame #15 {
                        n2315 = local read "Remarks :"() -> (w3382:string)
                        n2316 = Concatenate Strings("Remarks :" ("Content"), w3382) -> (w3383:string)
                        n2317 = local read "EVENT LOG"() -> (w3386:string)
                        n2318 = call "Event Log.vi"("Content"=w3383, "EVENT LOG"=w3386) -> ("EVENT LOG"=w3385:string)  [unwired: 8 in, 1 out]
                        n2319 = local write "EVENT LOG"(w3385) -> ()
                      }
                      frame #16 {
                        n2320 = Wait (ms)(milliseconds to wait=u32 50) -> ()  [unwired: 1 out]
                      }
                      frame #17 {
                        n2321 = local read "USER ID"() -> (w3388:string)
                        n2322 = Concatenate Strings("Operator ID :" ("Content"), w3388) -> (w3390:string)
                        n2323 = local read "EVENT LOG"() -> (w3392:string)
                        n2324 = call "Event Log.vi"("Content"=w3390, "EVENT LOG"=w3392) -> ("EVENT LOG"=w3391:string)  [unwired: 8 in, 1 out]
                        n2325 = local write "EVENT LOG"(w3391) -> ()
                      }
                      frame #18 {
                        n2326 = Wait (ms)(milliseconds to wait=u32 50) -> ()  [unwired: 1 out]
                      }
                      frame #19 {
                        n2327 = disable-structure shown="Disabled" {
                          frame Disabled {
                            n2328 = local read "EVENT LOG"() -> (w3396:string)
                            n2329 = call "Event Log.vi"("Content"="Test Parameter", "EVENT LOG"=w3396) -> ("EVENT LOG"=w3395:string)  [unwired: 8 in, 1 out]
                            n2330 = local write "EVENT LOG"(w3395) -> ()
                          }
                          frame Enabled {
                          }
                        }
                      }
                      frame #20 {
                        n2331 = Wait (ms)(milliseconds to wait=u32 50) -> ()  [unwired: 1 out]
                      }
                      frame #21 {
                        n2332 = local read "Set Hz"() -> (w3400:dbl)
                        n2333 = Number To Fractional String(number=w3400, precision (6)=i16 2) -> (F-format string=w3399:string)  [unwired: 2 in]
                        n2334 = Concatenate Strings("Set Frequency [Hz] :" ("Content"), w3399) -> (w3402:string)
                        n2335 = local read "EVENT LOG"() -> (w3404:string)
                        n2336 = call "Event Log.vi"("Content"=w3402, "EVENT LOG"=w3404) -> ("EVENT LOG"=w3403:string)  [unwired: 8 in, 1 out]
                        n2337 = local write "EVENT LOG"(w3403) -> ()
                      }
                      frame #22 {
                        n2338 = Wait (ms)(milliseconds to wait=u32 50) -> ()  [unwired: 1 out]
                      }
                      frame #23 {
                        n2339 = local read "NORMAL LOAD"() -> (w3407:dbl)
                        n2340 = Number To Fractional String(number=w3407, precision (6)=i16 2) -> (F-format string=w3408:string)  [unwired: 2 in]
                        n2341 = Concatenate Strings("Applied Load [grams] :" ("Content"), w3408) -> (w3410:string)
                        n2342 = local read "EVENT LOG"() -> (w3412:string)
                        n2343 = call "Event Log.vi"("Content"=w3410, "EVENT LOG"=w3412) -> ("EVENT LOG"=w3411:string)  [unwired: 8 in, 1 out]
                        n2344 = local write "EVENT LOG"(w3411) -> ()
                      }
                      frame #24 {
                        n2345 = Wait (ms)(milliseconds to wait=u32 50) -> ()  [unwired: 1 out]
                      }
                      frame #25 {
                        n2346 = local read "Set Strk"() -> (w3415:dbl)
                        n2347 = Number To Fractional String(number=w3415, precision (6)=i16 2) -> (F-format string=w3416:string)  [unwired: 2 in]
                        n2348 = Concatenate Strings("Set Stroke [mm] :" ("Content"), w3416) -> (w3418:string)
                        n2349 = local read "EVENT LOG"() -> (w3420:string)
                        n2350 = call "Event Log.vi"("Content"=w3418, "EVENT LOG"=w3420) -> ("EVENT LOG"=w3419:string)  [unwired: 8 in, 1 out]
                        n2351 = local write "EVENT LOG"(w3419) -> ()
                      }
                      frame #26 {
                        n2352 = Wait (ms)(milliseconds to wait=u32 50) -> ()  [unwired: 1 out]
                      }
                      frame #27 {
                        n2353 = local read "Set Temp"() -> (w3423:dbl)
                        n2354 = Number To Fractional String(number=w3423, precision (6)=i16 2) -> (F-format string=w3424:string)  [unwired: 2 in]
                        n2355 = Concatenate Strings("Set Temperature [deg C] :" ("Content"), w3424) -> (w3426:string)
                        n2356 = local read "EVENT LOG"() -> (w3428:string)
                        n2357 = call "Event Log.vi"("Content"=w3426, "EVENT LOG"=w3428) -> ("EVENT LOG"=w3427:string)  [unwired: 8 in, 1 out]
                        n2358 = local write "EVENT LOG"(w3427) -> ()
                      }
                      frame #28 {
                        n2359 = Wait (ms)(milliseconds to wait=u32 50) -> ()  [unwired: 1 out]
                      }
                      frame #29 {
                        n2360 = local read "Set Rh"() -> (w3431:dbl)
                        n2361 = Number To Fractional String(number=w3431, precision (6)=i16 2) -> (F-format string=w3432:string)  [unwired: 2 in]
                        n2362 = Concatenate Strings("Set Humidity [%RH] :" ("Content"), w3432) -> (w3434:string)
                        n2363 = local read "EVENT LOG"() -> (w3436:string)
                        n2364 = call "Event Log.vi"("Content"=w3434, "EVENT LOG"=w3436) -> ("EVENT LOG"=w3435:string)  [unwired: 8 in, 1 out]
                        n2365 = local write "EVENT LOG"(w3435) -> ()
                      }
                      frame #30 {
                        n2366 = Wait (ms)(milliseconds to wait=u32 50) -> ()  [unwired: 1 out]
                      }
                      frame #31 {
                        n2367 = local read "test time"() -> (w3439:dbl)
                        n2368 = Number To Fractional String(number=w3439, precision (6)=i16 1) -> (F-format string=w3440:string)  [unwired: 2 in]
                        n2369 = Concatenate Strings("Test Duration [mins] :" ("Content"), w3440) -> (w3442:string)
                        n2370 = local read "EVENT LOG"() -> (w3444:string)
                        n2371 = call "Event Log.vi"("Content"=w3442, "EVENT LOG"=w3444) -> ("EVENT LOG"=w3443:string)  [unwired: 8 in, 1 out]
                        n2372 = local write "EVENT LOG"(w3443) -> ()
                      }
                      frame #32 {
                        w3445 = dbl[] [] ("History Data")
                        w3446 = cluster{"y":dbl, dbl, "y":dbl}[] [] ("History Data")
                        w3447 = FALSE ("Visible")
                        n2373 = property on="Stroke ( mm )" class="WFChart (strict)"("History Data"=w3446) -> ()  [unwired: 2 in, 2 out]
                        n2374 = property on="Humidity ( %RH )" class="WFChart (strict)"("History Data"=w3445) -> ()  [unwired: 2 in, 2 out]
                        n2375 = property on="Temperature ( Deg C )" class="WFChart (strict)"("History Data"=w3445) -> ()  [unwired: 2 in, 2 out]
                        n2376 = property on="Electrical Contact Resistance ( % )" class="WFChart (strict)"("History Data"=w3445) -> ()  [unwired: 2 in, 2 out]
                        n2377 = property on="Coefficient of Friction" class="WFChart (strict)"("History Data"=w3445) -> ()  [unwired: 2 in, 2 out]
                        n2378 = property on="Frictional Force ( N )" class="WFChart (strict)"("History Data"=w3445) -> ()  [unwired: 2 in, 2 out]
                        n2379 = property on="Coefficient of Friction" class="WFChart (strict)"("History Data"=w3445) -> ()  [unwired: 2 in, 2 out]
                        n2380 = property on="Frictional Force ( N )" class="WFChart (strict)"("History Data"=w3445) -> ()  [unwired: 2 in, 2 out]
                        n2381 = property on="Electrical Contact Resistance ( % )" class="WFChart (strict)"("History Data"=w3445) -> ()  [unwired: 2 in, 2 out]
                        n2382 = property on="Humidity ( %RH )" class="WFChart (strict)"("History Data"=w3445) -> ()  [unwired: 2 in, 2 out]
                        n2383 = property on="Stroke ( mm )" class="WFChart (strict)"("History Data"=w3446) -> ()  [unwired: 2 in, 2 out]
                        n2384 = property on="Temperature ( Deg C )" class="WFChart (strict)"("History Data"=w3445) -> ()  [unwired: 2 in, 2 out]
                        n2385 = property on="Service Password Log" class="Str"("Visible"=w3447) -> ()  [unwired: 2 in, 2 out]
                        n2386 = property on="Password 3" class="Clust (strict)"("Visible"=w3447) -> ()  [unwired: 2 in, 2 out]
                      }
                    }
                    "TEST FILE NAM,E SAVED" <- TRUE ("TEST FILE NAM,E SAVED")
                  }
                }
              }
            }
          }
        }
        n2387 = local write "Test \nStatus"(w2837) -> ()
        n2388 = local write "Save"(w2837) -> ()
        n2389 = local read "Main Tab"() -> (w2831:T2)
        n2390 = case shown="True" w2834 {
          frame False {
            n2391 = local read "Rt 3"() -> (w2906:bool)
            n2392 = case shown="True" w2906 {
              frame False {
              }
              frame True {
                n2393 = local write "Rt 3"(FALSE ("Rt 3")) -> ()
              }
            }
            "Rt" <- TRUE ("Rt")
            "Rt 2" <- FALSE ("Rt")
          }
          frame True {
            n2394 = local read "Rt"() -> (w2912:bool)
            n2395 = local write "Rt 2"(TRUE ("Rt 2")) -> ()
            n2396 = case shown="True" w2912 {
              frame False {
              }
              frame True {
                n2397 = local write "Rt"(FALSE ("Rt")) -> ()
              }
            }
            "Rt 3" <- TRUE ("Rt 3")
          }
        }
        n2398 = case shown="\"Acquire\"" w2831 {
          tunnel: w2833 -> [_ w2940]
          frame Default {
            w2939 = 0.0 ("output")
            n2399 = local write "PID-out"(w2939) -> ()
            n2400 = local write "Frequency ( Hz )"(w2939) -> ()
          }
          frame "Acquire" {
            n2401 = stacked-sequence {
              frame #0 {
                n2402 = local read "Auto Start Test"() -> (w2942:bool)
                n2403 = case shown="True" w2942 {
                  tunnel: "RUN" -> [w2963 w2966]
                  tunnel: [w2963 w2965] -> w2943
                  frame False {
                  }
                  frame True {
                    n2404 = local read "Auto Start Temp"() -> (w2964:bool)
                    n2405 = Or(x=w2966, y=w2964) -> (x .or. y?=w2965:bool)
                  }
                }
                n2406 = local read "clk"() -> (w2962:dbl)
                n2407 = local read "Save"() -> (w2958:bool)
                n2408 = Equal?(x=w2962, y=0.0) -> (x = y?=w2959:bool)
